vi "broadcastHPSteps.vi"(8 "error in (no error)":errorcluster, 9 "TriggerIRQ":bool, 10 "WaitForTrigger":bool, 11 "ILCCommunications in":refnum<class "ILCCommunications.lvclass">) -> (0 "error out":errorcluster, 3 "ILCCommunications out":refnum<class "ILCCommunications.lvclass">)   [LabVIEW 2016, in "ILCCommunications.lvclass"]
uses:
  ILCCommunications.lvclass
  ILCCommunications.lvclass/ILCCommunications.ctl
  Common_RT_Modbus/IModbus/IModbus.lvclass
  Common_RT_HPILC/HPILC/HPILC.lvclass
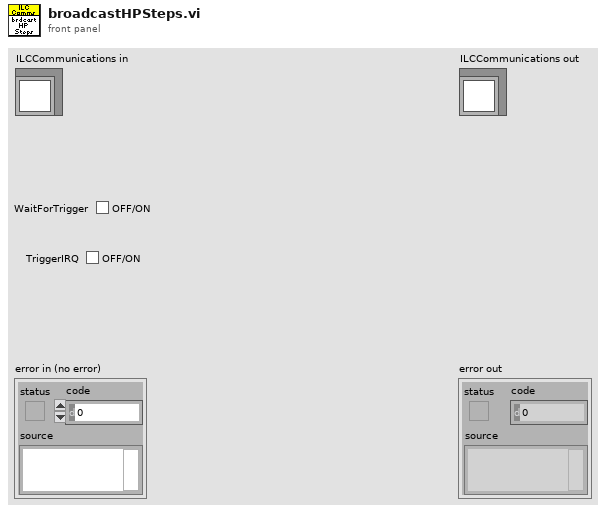
[diagram p1: front panel]
types:
  T1 = typedef "RTModbus.lvlib/TxFrame.ctl" = cluster{"Data":u8[], "WaitForTrigger":bool, "WaitForRx":u16, "TriggerIRQ":bool, "DelayMicroseconds":u16, "DelayMilliseconds":u16, "Timestamp":bool}
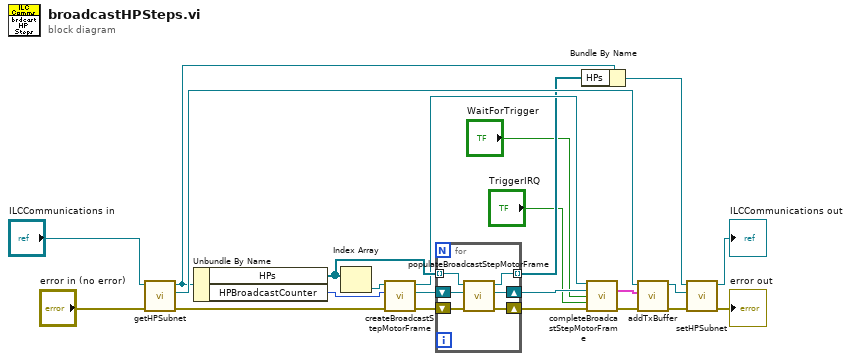
[diagram p0: block diagram]
diagram:
  n1 = call "getHPSubnet.vi"("error in (no error)"="error in (no error)", "ILCCommunications in"="ILCCommunications in") -> ("error out"=w13:errorcluster, "Modbus"=w11:refnum<class "IModbus.lvclass">, "ILCCommunications out"=w5:refnum<class "ILCCommunications.lvclass">)  [unwired: 7 in]
  n2 = Unbundle By Name(w5) -> ("HPs"=w20:refnum<class "HPILC.lvclass">[], "HPBroadcastCounter"=w22:u8)
  n3 = Index Array(array=w20) -> (element=w21:refnum<class "HPILC.lvclass">)  [unwired: 1 in]
  n4 = call "createBroadcastStepMotorFrame.vi"("error in (no error)"=w13, "BroadcastCounter"=w22, "HPILC in"=w21) -> ("error out"=w18:errorcluster, "FixedFrameBuilder"=w19:refnum<class "FixedFrameBuilder.lvclass">, "HPILC out"=w17:refnum<class "HPILC.lvclass">)  [unwired: 6 in]
  n5 = for {
    tunnel: w20 -> [w29] mode=indexing
    shift-right: [w27] -> w16
    shift-left: w19 -> [w28]
    tunnel: [w26] -> w3 mode=indexing
    shift-right: [w24] -> w15
    shift-left: w18 -> [w25]
    n6 = call "populateBroadcastStepMotorFrame.vi"("error in (no error)"=w25, "FixedFrameBuilder in"=w28, "HPILC in"=w29) -> ("error out"=w24:errorcluster, "FixedFrameBuilder out"=w27:refnum<class "FixedFrameBuilder.lvclass">, "HPILC out"=w26:refnum<class "HPILC.lvclass">)  [unwired: 6 in]
  }
  n7 = Bundle By Name(cluster=w5, "HPs"=w3) -> (w4:refnum<class "ILCCommunications.lvclass">)
  n8 = call "completeBroadcastStepMotorFrame.vi"("HPILC in"=w17, "FixedFrameBuilder"=w16, "WaitForTrigger"="WaitForTrigger", "TriggerIRQ"="TriggerIRQ", "error in (no error)"=w15) -> ("TxFrame"=w12:T1, "error out"=w9:errorcluster)  [unwired: 8 in, 1 out]
  n9 = call-dynamic "addTxBuffer.vi"("error in (no error)"=w9, "TxFrame"=w12, "IModbus in"=w11) -> ("error out"=w7:errorcluster, "IModbus out"=w10:refnum<class "IModbus.lvclass">)  [unwired: 7 in]
  n10 = call "setHPSubnet.vi"("error in (no error)"=w7, "Modbus"=w10, "ILCCommunications in"=w4) -> ("error out"=→"error out":errorcluster, "ILCCommunications out"=→"ILCCommunications out":refnum<class "ILCCommunications.lvclass">)  [unwired: 7 in]
